vi "_tester3_.vi"() -> ()   [LabVIEW 2025]
uses:
  LabVIEWpcm.dll
panel:
  out "Iteration Time":dbl(graph)
  out "IPC":dbl(graph)
  in  "F = ROW, T = COL":bool=TRUE
  out "sum":u8
  in  "Stop Button":bool
  out "counrters":i32
  out "Level 3 Miss":u64(graph)
  out "Level 3 Hit":dbl(graph)
  out "Level 2 miss":u64(graph)
  out "Level 2 Hit":dbl(graph)
  out "init":i32
  # "MUST BE RUN AS ADMINISTRATOR!!!"
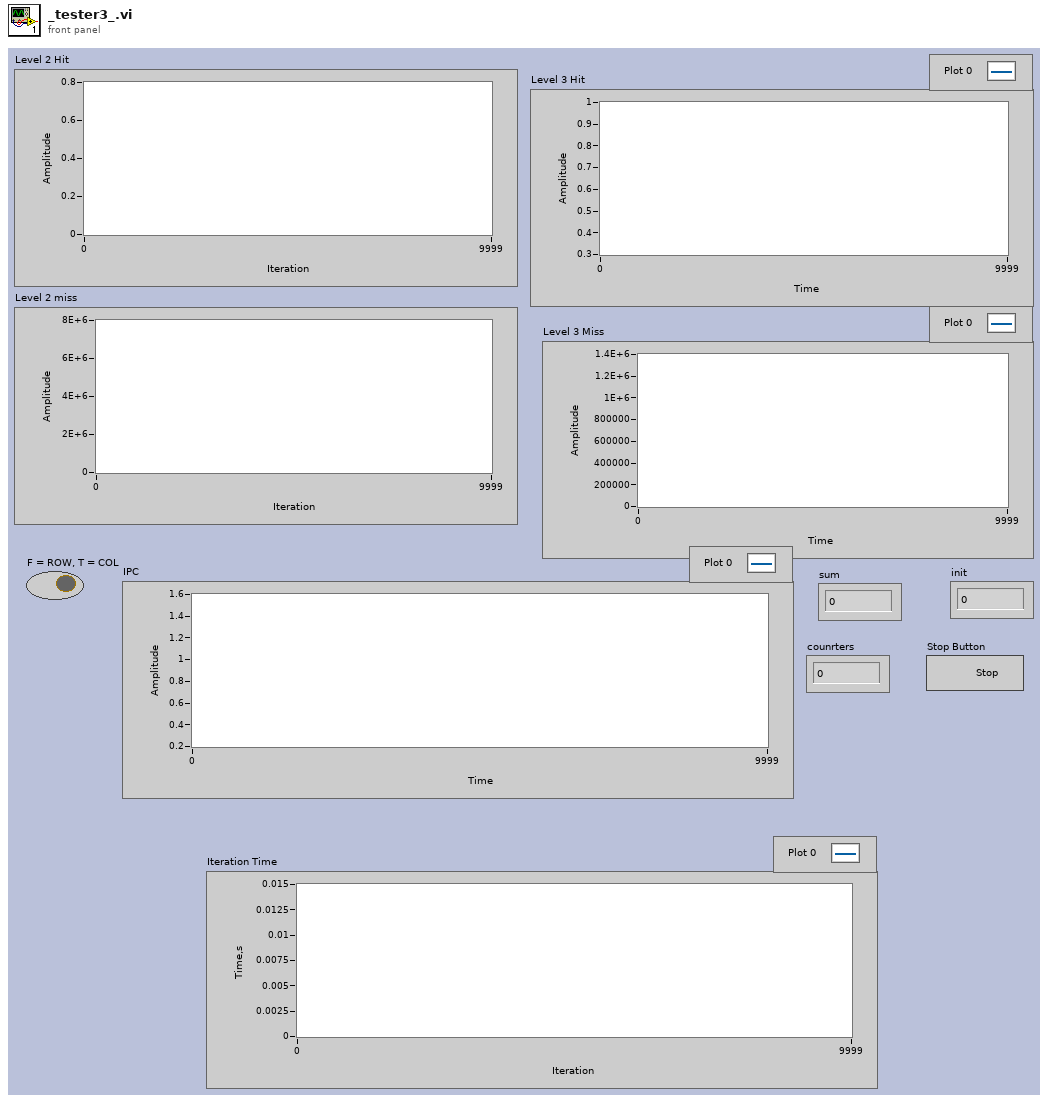
[diagram p1: front panel]
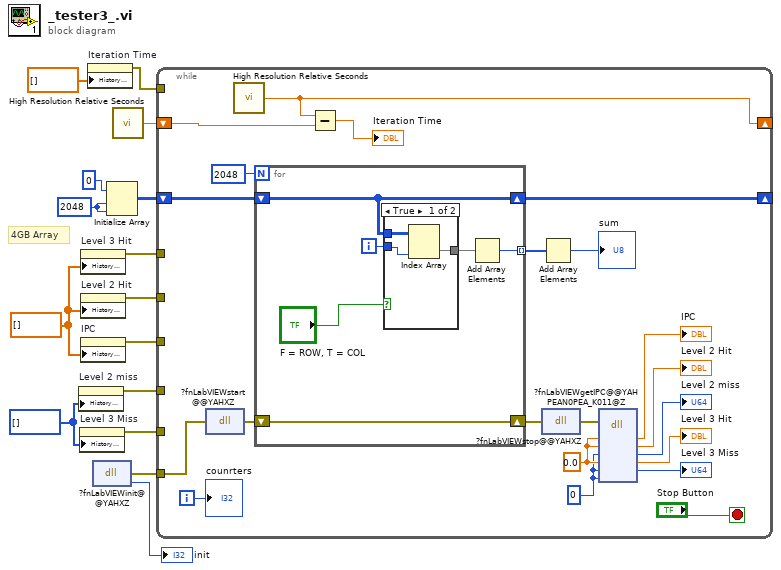
[diagram p0: block diagram]
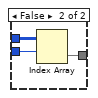
[diagram p2: hidden frame]
diagram:
  w9 = u64[] [] ("History Data")
  w10 = dbl[] [] ("History Data")
  w12 = 2048 ("dimension size")
  # "4GB Array"
  n1 = property on="Level 2 miss" class="WFChart (strict)"("History Data"=w9) -> (error out=w6:errorcluster)  [unwired: 2 in, 1 out]
  n2 = property on="Level 3 Miss" class="WFChart (strict)"("History Data"=w9) -> (error out=w4:errorcluster)  [unwired: 2 in, 1 out]
  n3 = property on="Level 3 Hit" class="WFChart (strict)"("History Data"=w10) -> (error out=w5:errorcluster)  [unwired: 2 in, 1 out]
  n4 = property on="Level 2 Hit" class="WFChart (strict)"("History Data"=w10) -> (error out=w7:errorcluster)  [unwired: 2 in, 1 out]
  n5 = property on="IPC" class="WFChart (strict)"("History Data"=w10) -> (error out=w8:errorcluster)  [unwired: 2 in, 1 out]
  n6 = property on="Iteration Time" class="WFChart (strict)"("History Data"=dbl[] []) -> (error out=w1:errorcluster)  [unwired: 2 in, 1 out]
  n7 = dll-call lib="C:/Users/Andrey/Desktop/intel-pcm/build/x64/Release/LabVIEWpcm.dll" fn="?fnLabVIEWinit@@YAHXZ"() -> (error out=w15:errorcluster, "return type"=→"init":i32)  [unwired: 3 in, 1 out]
  n8 = Initialize Array(u8 0, w12, w12) -> (w11:u8[][])
  n9 = call <vilib>:"High Resolution Relative Seconds.vi"() -> ("relative seconds"=w3:dbl)
  n10 = while {
    tunnel: w15 -> [w36]
    shift-right: [w22] -> _
    shift-left: w11 -> [w23]
    tunnel: w8 -> [_]
    tunnel: w7 -> [_]
    tunnel: w6 -> [_]
    tunnel: w5 -> [_]
    tunnel: w4 -> [_]
    shift-right: [w17] -> _
    shift-left: w3 -> [w18]
    tunnel: w1 -> [_]
    i -> [w28]
    stop <- "Stop Button" stop-if-true
    w33 = u64 0 ("bytes")
    w34 = 0.0 ("ipc")
    n11 = dll-call lib="C:/Users/Andrey/Desktop/intel-pcm/build/x64/Release/LabVIEWpcm.dll" fn="?fnLabVIEWstart@@YAHXZ"(error in=w36) -> (error out=w20:errorcluster)  [unwired: 3 in, 1 out]
    n12 = call <vilib>:"High Resolution Relative Seconds.vi"() -> ("relative seconds"=w17:dbl)
    n13 = for {
      N: 2048 ("dimension size") -> [_]
      tunnel: [w41] -> w25 mode=indexing
      shift-right: [w40] -> w22
      shift-left: w23 -> [w40]
      shift-right: [w39] -> w21
      shift-left: w20 -> [w39]
      i -> [w38]
      n14 = case shown="True" "F = ROW, T = COL" {
        tunnel: [w45 w48] -> w42
        tunnel: w40 -> [w44 w47]
        tunnel: w38 -> [w43 w46]
        frame True {
          n15 = Index Array(array=w44, index (col)=w43) -> (element=w45:u8[])  [unwired: 1 in]
        }
        frame False {
          n16 = Index Array(array=w47, index (row)=w46) -> (element=w48:u8[])  [unwired: 1 in]
        }
      }
      n17 = Add Array Elements(numeric array=w42) -> (sum=w41:u8)
    }
    n18 = Subtract(x=w17, y=w18) -> (x-y=→"Iteration Time":dbl)
    n19 = dll-call lib="C:/Users/Andrey/Desktop/intel-pcm/build/x64/Release/LabVIEWpcm.dll" fn="?fnLabVIEWstop@@YAHXZ"(error in=w21) -> (error out=w35:errorcluster)  [unwired: 3 in, 1 out]
    n20 = Add Array Elements(numeric array=w25) -> (sum=→"sum":u8)
    n21 = dll-call lib="C:/Users/Andrey/Desktop/intel-pcm/build/x64/Release/LabVIEWpcm.dll" fn="?fnLabVIEWgetIPC@@YAHPEAN0PEA_K011@Z"(error in=w35, "ipc"=w34, "lv2hit"=w34, "lv2miss"=w33, "l3hit"=w34, "l3miss"=w33, "bytes"=w33) -> ("ipc"=→"IPC":dbl, "lv2hit"=→"Level 2 Hit":dbl, "lv2miss"=→"Level 2 miss":u64, "l3hit"=→"Level 3 Hit":dbl, "l3miss"=→"Level 3 Miss":u64)  [unwired: 4 in, 2 out]
    "counrters" <- w28
  }
